vi "DSF.Engine.Transceiver.Initialize.vi"(8 "error in (no error)":errorcluster, 9 "transceiver settings":T1, 10 "Transfer Groups Configurations":refnum<class "Transfer Group Configuration.lvclass">[](array[class]), 11 "UDP Transceiver in":refnum<class "DSF.Transceiver.UDP.lvclass">=refnum) -> (0 "error out":errorcluster, 3 "UDP Transceiver out":refnum<class "DSF.Transceiver.UDP.lvclass">)   [LabVIEW 2017, in "DSF.Transceiver.UDP.lvlib" / "DSF.Transceiver.UDP.lvclass"]
uses:
  DSF.Transceiver.UDP.lvclass
  Builds/Current/Data Sharing Framework Core/Data Sharing Framework Core.lvlibp/Engine/Internal/Configuration Classes/Transfer Group Configuration/Transfer Group Configuration.lvclass
  C:/github/data-sharing-framework/Builds/Current/Data Sharing Framework Core/Data Sharing Framework Core.lvlibp/Engine/Internal/Configuration Classes/Configuration/Configuration.lvclass
  DSF Core/Built/Engine/DSF.Engine.lvlibp/DSF Configuration API/1.0.0/Public/Controls/DSF Settings Info.ctl
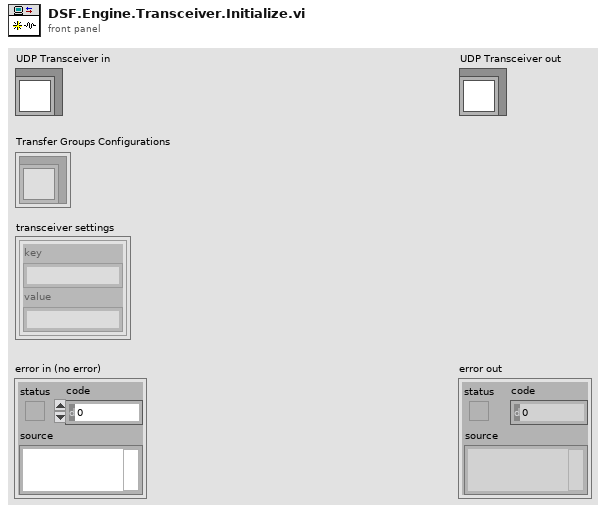
[diagram p1: front panel]
types:
  T1 = typedef "DSF.Engine.lvlibp/DSF Configuration API.lvlib/DSF Settings Info.ctl" = cluster{"key":string, "value":string}[]
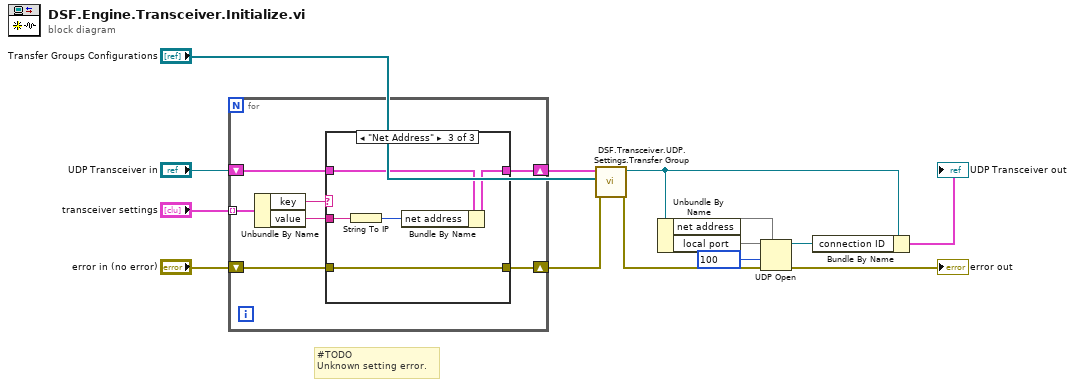
[diagram p0: block diagram]
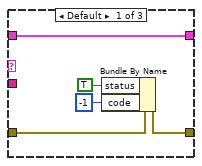
[diagram p2: hidden frame]
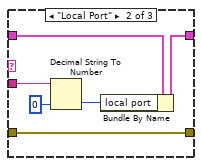
[diagram p3: hidden frame]
diagram:
  # "#TODO\nUnknown setting error."
  n1 = for {
    tunnel: "transceiver settings" -> [w21] mode=indexing
    shift-right: [w17] -> w12
    shift-left: "UDP Transceiver in" -> [w18]
    shift-right: [w15] -> w10
    shift-left: "error in (no error)" -> [w16]
    n2 = Unbundle By Name(w21) -> ("key"=w20:string, "value"=w19:string)
    n3 = case shown="\"Net Address\"" w20 {
      tunnel: w19 -> [_ w31 w34]
      tunnel: w18 -> [w26 w30 w37]
      tunnel: [w26 w29 w36] -> w17
      tunnel: w16 -> [w25 w28 w35]
      tunnel: [w24 w28 w35] -> w15
      frame Default {
        n4 = Bundle By Name(cluster=w25, "status"=TRUE, "code"=-1) -> (w24:errorcluster)
      }
      frame "Local Port" {
        n5 = Decimal String To Number(string=w31, default (0L)=u16 0 ("default (0 I32)")) -> (number=w27:u16)  [unwired: 1 in, 1 out]
        n6 = Bundle By Name(cluster=w30, "local port"=w27) -> (w29:cluster{})
      }
      frame "Net Address" {
        n7 = String To IP(1:w34) -> (0:w33:u32)
        n8 = Bundle By Name(cluster=w37, "net address"=w33) -> (w36:cluster{})
      }
    }
  }
  n9 = call "DSF.Transceiver.UDP.Settings.Transfer Group.vi"("error in (no error)"=w10, "Transfer Groups Configurations"="Transfer Groups Configurations", "UDP Transceiver in"=w12) -> ("error out"=w9:errorcluster, "UDP Transceiver out"=w8:refnum<class "DSF.Transceiver.UDP.lvclass">)  [unwired: 7 in]
  n10 = Unbundle By Name(w8) -> ("net address"=w2, "local port"=w7)
  n11 = UDP Open(7:w2, 8:w9, 9:100 ("timeout ms (25000)"), 11:w7) -> (port=w5:refnum<k16>, 0:→"error out":errorcluster)  [unwired: 1 in, 1 out]
  n12 = Bundle By Name(cluster=w8, "connection ID"=w5) -> (→"UDP Transceiver out":cluster{})
